vi "PasteSelectedCells.vi"(4 "ModeCol Index":i32=2, 5 "Layout Ref":refnum<vi>, 6 "Clipboard":refnum<vi>, 7 "Table History ref":refnum<vi>, 8 "error in (no error)":errorcluster, 9 "Table CtlRef In":refnum<vi>, 10 "Cell Start":T1, 11 "Col Array Ref in":refnum<vi>) -> (0 "error out":errorcluster, 1 "Table CtlRef Out":refnum<vi>, 3 "Col Array Ref out":refnum<vi>)   [LabVIEW 2013]
doc: "\"Safely\" paste clipboard into selection, first coercing the data (with user warning) so that it fits within the table lines.\nThis VI is read-only w.r.t column data."
uses:
  <vilib>/Utility/miscctls.llb/LVRowAndColumnTypeDef.ctl
  TypeDefs/TableHistory.ctl
  TypeDefs/TableArray.ctl
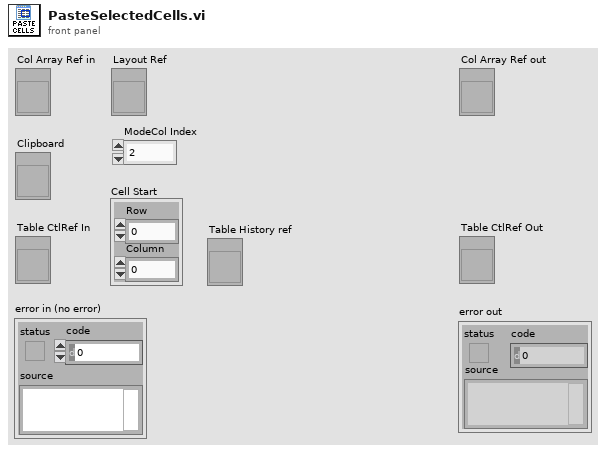
[diagram p1: front panel]
types:
  T1 = typedef "LVRowAndColumnTypeDef.ctl" = cluster{"Row":i32, "Column":i32}
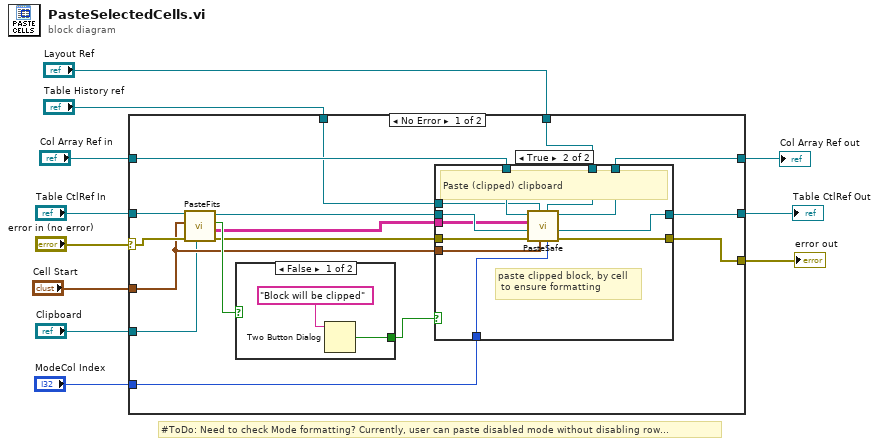
[diagram p0: block diagram]
diagram:
  # "#ToDo: Need to check Mode formatting? Currently, user can paste disabled mode without disabling row..."
  n1 = case shown="No Error" "error in (no error)" {
    selector: "error in (no error)" -> [w20 w46]
    tunnel: "Table CtlRef In" -> [w21 w47]
    tunnel: "Clipboard" -> [w15 _]
    tunnel: [w22 w47] -> w9
    tunnel: [w19 w46] -> w8
    tunnel: [w18 w45] -> w6
    tunnel: "Col Array Ref in" -> [w17 w45]
    tunnel: "Cell Start" -> [w16 _]
    tunnel: "Table History ref" -> [w14 _]
    tunnel: "ModeCol Index" -> [w13 _]
    tunnel: "Layout Ref" -> [w12 _]
    frame No Error {
      n2 = call "PasteFits.vi"("Clipboard"=w15, "error in (no error)"=w20, "Cell Start"=w16, "Table CtlRef In"=w21) -> ("error out"=w26:errorcluster, "Clipboard (clipped)"=w24:string[][], "Paste Fits?"=w27:bool, "Table CtlRef Out"=w25:refnum<vi>)  [unwired: 4 in]
      n3 = case shown="False" w27 {
        selector: w27 -> [_ w44]
        tunnel: [w43 w44] -> w23
        frame False {
          n4 = Two Button Dialog(message="Block will be clipped") -> (T button?=w43:bool)  [unwired: 2 in]
        }
        frame True {
        }
      }
      n5 = case shown="True" w23 {
        tunnel: w26 -> [w28 w41]
        tunnel: [w28 w40] -> w19
        tunnel: w25 -> [w29 w39]
        tunnel: [w29 w38] -> w22
        tunnel: w17 -> [w30 w37]
        tunnel: [w30 w36] -> w18
        tunnel: w24 -> [_ w35]
        tunnel: w16 -> [_ w34]
        tunnel: w14 -> [_ w33]
        tunnel: w13 -> [_ w32]
        tunnel: w12 -> [_ w31]
        frame False {
          # "User cancelled due to clipping"
        }
        frame True {
          # "paste clipped block, by cell\n to ensure formatting"
          # "Paste (clipped) clipboard"
          n6 = call "PasteSafe.vi"("ModeCol Index"=w32, "Layout Ref"=w31, "Cell Start"=w34, "Table History ref"=w33, "error in (no error)"=w41, "Table CtlRef In"=w39, "Clipboard (clipped)"=w35, "Col Array Ref in"=w37) -> ("error out"=w40:errorcluster, "Table CtlRef Out"=w38:refnum<vi>, "Col Array Ref out"=w36:refnum<vi>)  [unwired: 1 in]
        }
      }
    }
    frame Error {
    }
  }
  "error out" <- w8
  "Table CtlRef Out" <- w9
  "Col Array Ref out" <- w6
